vi "Averaged frame speed value.vi"(1 "Reshaped speed data array":dbl[](array[numeric])) -> (0 "Average value":dbl)   [LabVIEW 2013]
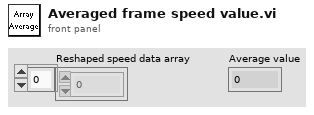
[diagram p1: front panel]
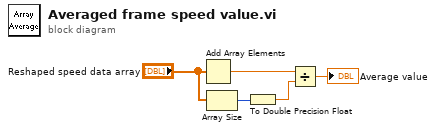
[diagram p0: block diagram]
diagram:
  n1 = Add Array Elements(numeric array="Reshaped speed data array") -> (sum=w3:dbl)
  n2 = Array Size(array="Reshaped speed data array") -> (size(s)=w4:i32)
  n3 = To Double Precision Float(number=w4) -> (double precision float=w1:dbl)
  n4 = Divide(x=w3, y=w1) -> (x/y=→"Average value":dbl)
